vi "Listening Server Cases.vi"(7 "Listening Queue":refnum<queue>, 8 "error in (no error)":errorcluster, 9 "Data":variant, 10 "Command":string, 11 "Generic Optimizer in":refnum<class "Generic Optimizer.lvclass">) -> (0 "error out":errorcluster, 2 "Stop?":bool, 3 "Generic Optimizer out":refnum<class "Generic Optimizer.lvclass">)   [LabVIEW 2020, in "RxnRover.lvlib" / "Generic Optimizer.lvclass"]
doc: "Case structure with messages to listen for from the control panel. If more than the basic messages need to be handled, this should be overwritten by the child class."
uses:
  Generic Optimizer.lvclass
  C:/Users/zachc/programs/rxnrover_workspace/rxnrover/src/RxnRover/Plugin Servers/Controller/Generic Plugin.lvclass
  <userlib>/RxnRover/DynamicReentrant/src/Type Defs/Message.ctl
  events/Process Stopped Cluster.ctl
  Controller/Generic Plugin.lvclass/Generic Plugin.ctl
  Sub VIs/Message Queue/Enqueue Message (Single).vi
  RxnRover.lvlib
  Sub VIs/Message Queue/test Message Queue.lvlib
  Controller/Generic Plugin.lvclass
  <userlib>/RxnRover/DynamicReentrant/Dynamic Reentrant.lvlib
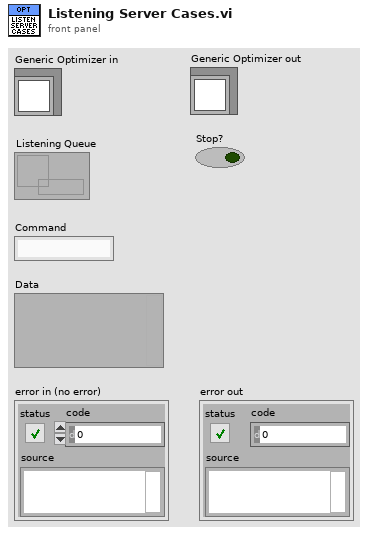
[diagram p1: front panel]
types:
  T1 = typedef "RxnRover.lvlib/Process Stopped Cluster.ctl" = cluster{"Name":string, "Type":enum16{"Hardware", "Optimizer", "Analyzer"}}
  T2 = typedef "RxnRover.lvlib/Generic Optimizer.lvclass/Generic Optimizer State.ctl" = cluster{"Running Since":timestamp, "New Parameters":cluster{"Time Stamp":timestamp, "Names":string[], "Values":dbl[]}, "Optimizer Path":path, "Running":bool}
  T3 = cluster{"Time Stamp":timestamp, "Names":string[], "Values":dbl[]}
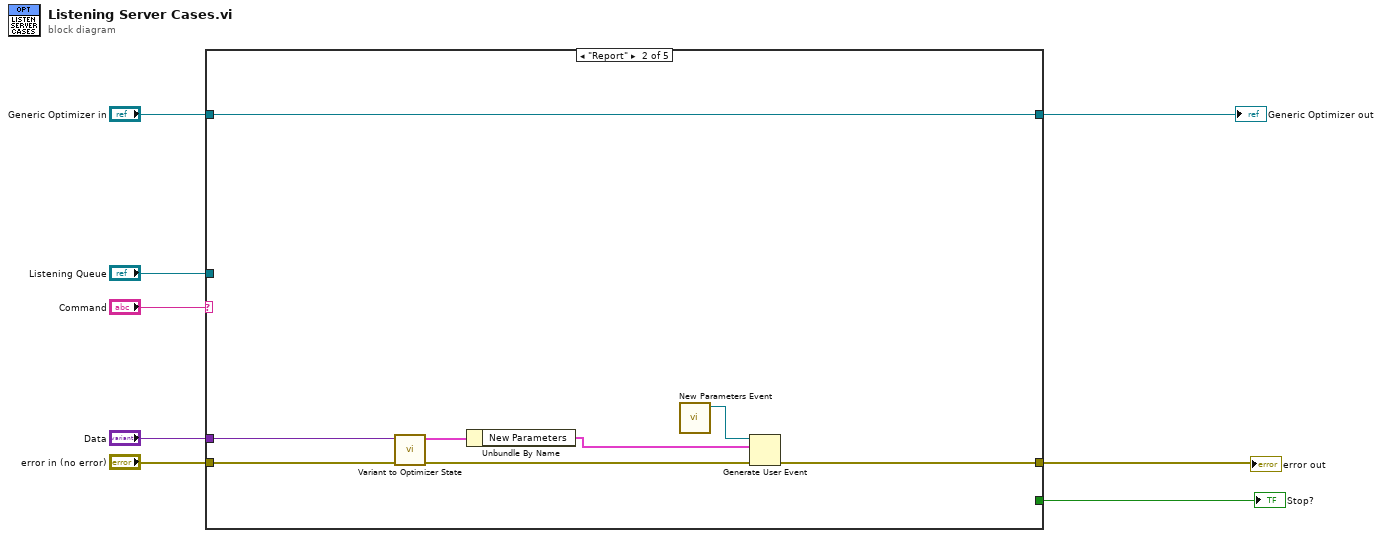
[diagram p0: block diagram]
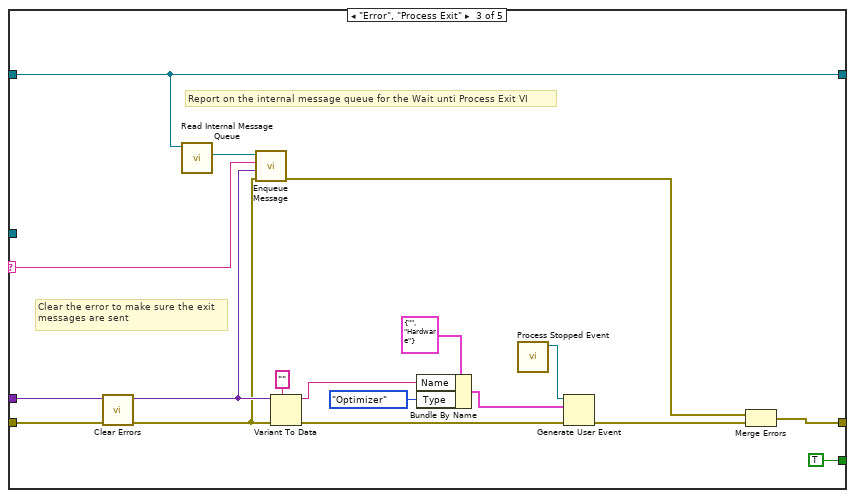
[diagram p3: hidden frame]
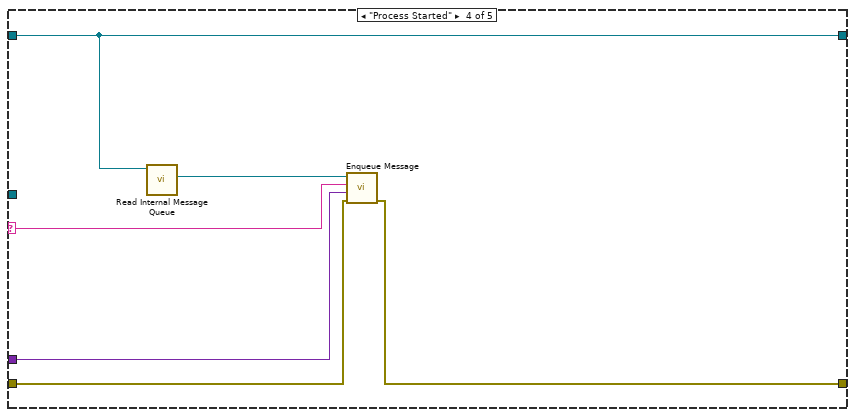
[diagram p4: hidden frame]
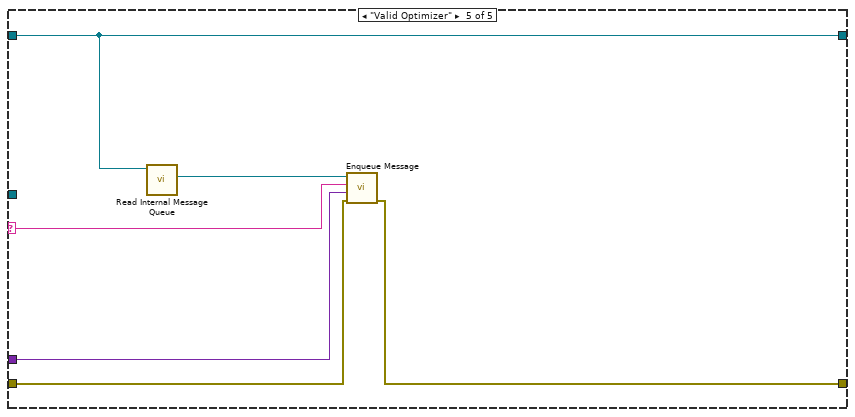
[diagram p5: hidden frame]
diagram:
  n1 = case shown="\"Report\"" "Command" {
    selector: "Command" -> [_ _ w23 w39 w45]
    tunnel: "error in (no error)" -> [w9 w13 w25 w37 w43]
    tunnel: [w9 w12 w22 w36 w42] -> w8
    tunnel: "Generic Optimizer in" -> [w10 w18 w20 w41 w47]
    tunnel: [w10 w18 w20 w41 w47] -> w6
    tunnel: "Data" -> [_ w11 w24 w38 w44]
    tunnel: [_ _ TRUE _ _] -> w7
    tunnel: "Listening Queue" -> [_ _ _ _ _]
    frame Default {
    }
    frame "Report" {
      n2 = call "Variant to Optimizer State.vi"("error in (no error)"=w13, "Message Data"=w11) -> ("error out"=w16:errorcluster, "Optimizer State"=w15:T2)  [unwired: 8 in]
      n3 = Unbundle By Name(w15) -> ("New Parameters"=w14:T3)
      n4 = call "New Parameters Event.vi"() -> ("New Parameters"=w17:refnum<user-event>)  [unwired: 11 in]
      n5 = Generate User Event(user event=w17, event data cluster=w14, error in=w16) -> (error out=w12:errorcluster)  [unwired: 1 in, 1 out]
    }
    frame "Error", "Process Exit" {
      # "Clear the error to make sure the exit\nmessages are sent"
      # "Report on the internal message queue for the Wait unti Process Exit VI"
      n6 = call <vilib>:"Clear Errors.vi"("error in (no error)"=w25) -> ("error out"=w19:errorcluster)  [unwired: 5 in, 1 out]
      n7 = call "Read Internal Message Queue.vi"("Generic Controller in"=w20) -> ("Internal Message Queue"=w26:refnum<queue>)  [unwired: 8 in, 2 out]
      n8 = call-poly "Enqueue Message.vi"("error in (no error)"=w19, "Message Data"=w24, "Message"=w23, "Message Queue"=w26) -> ("error out"=w21:errorcluster)  [unwired: 6 in, 1 out]
      n9 = Variant To Data(error in=w19, type="", Variant=w24) -> (data=w28:string, error out=w32:errorcluster)
      n10 = Bundle By Name(cluster=T1 {"Name"="", "Type"=enum."Hardware"} ("Process Cluster"), "Name"=w28, "Type"=enum16{"Hardware", "Optimizer"}."Optimizer") -> (w29:T1)
      n11 = call "Process Stopped Event.vi"() -> ("Process Stopped"=w34:refnum<user-event>)  [unwired: 11 in]
      n12 = Generate User Event(user event=w34, event data cluster=w29, error in=w32) -> (error out=w33:errorcluster)  [unwired: 1 in, 1 out]
      n13 = Merge Errors(w21, w33) -> (w22:errorcluster)
    }
    frame "Process Started" {
      n14 = call "Read Internal Message Queue.vi"("Generic Controller in"=w41) -> ("Internal Message Queue"=w40:refnum<queue>)  [unwired: 8 in, 2 out]
      n15 = call-poly "Enqueue Message.vi"("error in (no error)"=w37, "Message Data"=w38, "Message"=w39, "Message Queue"=w40) -> ("error out"=w36:errorcluster)  [unwired: 6 in, 1 out]
    }
    frame "Valid Optimizer" {
      n16 = call "Read Internal Message Queue.vi"("Generic Controller in"=w47) -> ("Internal Message Queue"=w46:refnum<queue>)  [unwired: 8 in, 2 out]
      n17 = call-poly "Enqueue Message.vi"("error in (no error)"=w43, "Message Data"=w44, "Message"=w45, "Message Queue"=w46) -> ("error out"=w42:errorcluster)  [unwired: 6 in, 1 out]
    }
  }
  "Stop?" <- w7
  "Generic Optimizer out" <- w6
  "error out" <- w8
